vi "计算桶探测器均值图像.vi"(0 "模块选择簇":T3, 5 "优化光源散斑簇":T2, 7 "图像信息簇":T1, 9 "散斑图像作用结果求和":dbl[](array[numeric]), 11 "散斑图像作用平均值":dbl) -> (4 "未归一化重建图像二维数组":dbl[][](array[numeric]))   [LabVIEW 2018]
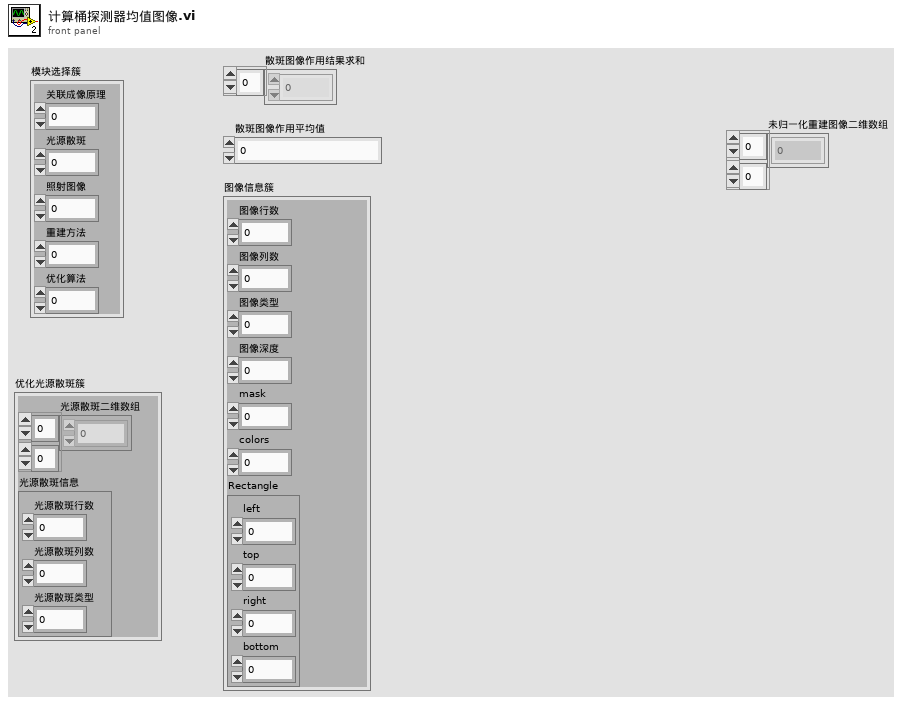
[diagram p1: front panel]
types:
  T1 = cluster{"图像行数":dbl, "图像列数":dbl, "图像类型":dbl, "图像深度":i32, "mask":i32, "colors":i32, "Rectangle":cluster{"left":i16, "top":i16, "right":i16, "bottom":i16}}
  T2 = cluster{"光源散斑二维数组":dbl[][], "光源散斑信息":cluster{"光源散斑行数":dbl, "光源散斑列数":dbl, "光源散斑类型":dbl}}
  T3 = cluster{"关联成像原理":i32, "光源散斑":i32, "照射图像":i32, "重建方法":i32, "优化算法":i32}
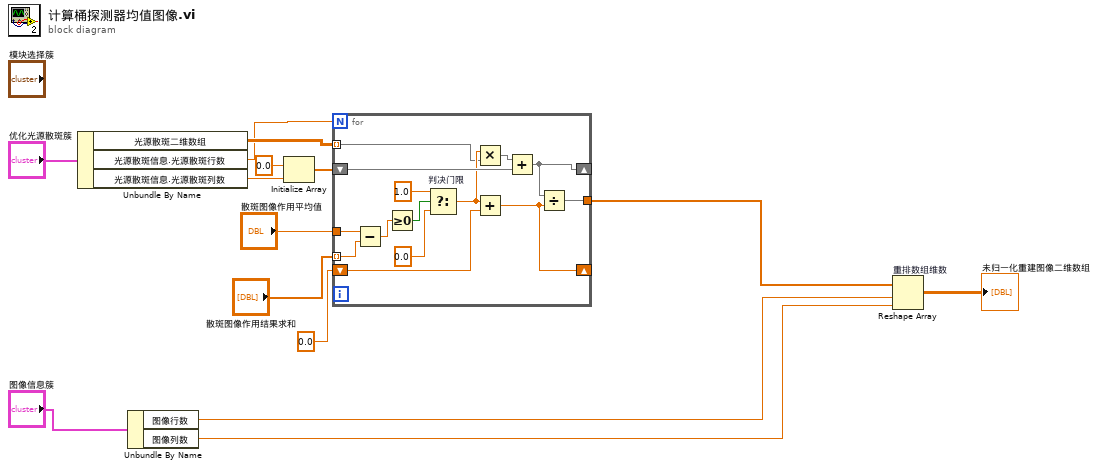
[diagram p0: block diagram]
diagram:
  n1 = Unbundle By Name("优化光源散斑簇") -> ("光源散斑二维数组"=w9:dbl[][], "光源散斑信息.光源散斑行数"=w8:dbl, "光源散斑信息.光源散斑列数"=w7:dbl)
  n2 = Unbundle By Name("图像信息簇") -> ("图像行数"=w3:dbl, "图像列数"=w2:dbl)
  n3 = Initialize Array ("1024长度的一维数组")(0.0 ("元素"), w7) -> (w13:dbl[])
  n4 = for {
    N: w8 -> [_]
    tunnel: "散斑图像作用平均值" -> [w18]
    tunnel: w9 -> [w16] mode=indexing
    shift-right: [w20] -> _
    shift-left: w13 -> [w23]
    shift-right: [w19] -> _
    shift-left: 0.0 ("元素") -> [w22]
    tunnel: "散斑图像作用结果求和" -> [w17] mode=indexing
    tunnel: [w15] -> w4
    n5 = Subtract(x=w18, y=w17) -> (x-y=w28:dbl)
    n6 = Greater Or Equal To 0?(x=w28) -> (x >= 0?=w27:bool)
    n7 = Select "判决门限"(t=1.0, s=w27, f=0.0) -> (s? t:f=w21:dbl)
    n8 = Multiply ("判决值和每行每个数相乘，导致某些行留下而某些行消失")(x=w21, y=w16) -> (x*y=w24:dbl[])
    n9 = Add(x=w21, y=w22) -> (x+y=w19:dbl)
    n10 = Add ("某些保留的行被突出和原始的相加")(x=w24, y=w23) -> (x+y=w20:dbl[])
    n11 = Divide(x=w20, y=w19) -> (x/y=w15:dbl[])
  }
  n12 = Reshape Array "重排数组维数"(w4, w3, w2) -> (→"未归一化重建图像二维数组":dbl[][])
